vi "Open Calibration Files.vi"(0 "Pressure Calibration Path":path, 1 "Estimated Tube Gain":dbl, 5 "Flow Array Path":path, 7 "SPL Calibration Path":path, 9 "operation (0:open)":T1(ring), 11 "error in (no error)":errorcluster, 12 "access (0:read/write)":enum16{"read/write", "read-only", "write-only"}(ring)) -> (3 "Pressure Slope":dbl, 4 "Pressure Intercept":dbl, 6 "Flow Array":dbl[](array[numeric]), 8 "Microphone Sensitivity":dbl, 10 "SPL Gain":dbl, 15 "error out":errorcluster)   [LabVIEW 2020, in "CollectionSupport.lvlib"]
uses:
  CollectionSupport.lvlib
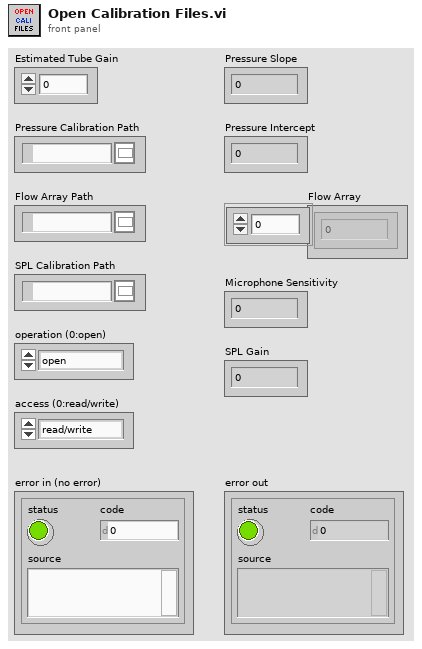
[diagram p1: front panel]
types:
  T1 = enum16{"open", "replace", "create", "open or create", "replace or create", "replace or create with confirmation"}
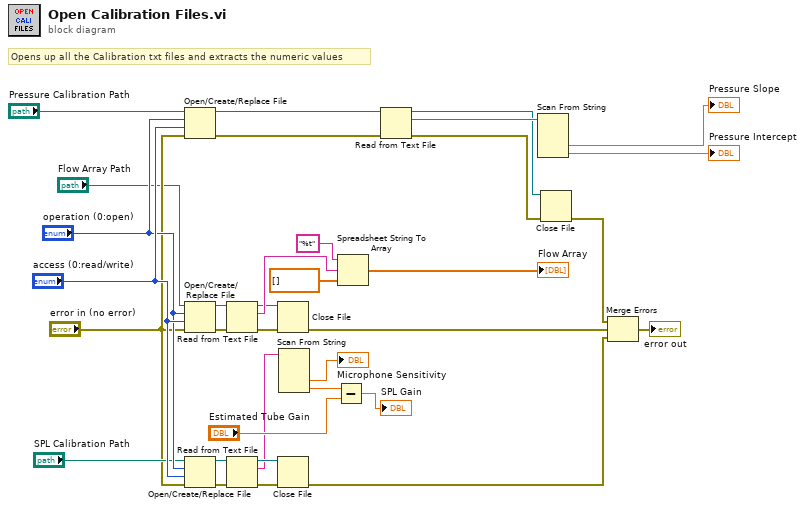
[diagram p0: block diagram]
diagram:
  # "Opens up all the Calibration txt files and extracts the numeric values"
  n1 = Open/Create/Replace File(file path (use dialog)="Pressure Calibration Path", error in="error in (no error)", operation (0:open)="operation (0:open)", access (0:read/write)="access (0:read/write)") -> (refnum out=w3:refnum<file>, error out=w1:errorcluster)  [unwired: 2 in, 1 out]
  n2 = Open/Create/Replace File(file path (use dialog)="Flow Array Path", error in="error in (no error)", operation (0:open)="operation (0:open)", access (0:read/write)="access (0:read/write)") -> (refnum out=w10:refnum<file>, error out=w8:errorcluster)  [unwired: 2 in, 1 out]
  n3 = Open/Create/Replace File(file path (use dialog)="SPL Calibration Path", error in="error in (no error)", operation (0:open)="operation (0:open)", access (0:read/write)="access (0:read/write)") -> (refnum out=w20:refnum<file>, error out=w22:errorcluster)  [unwired: 2 in, 1 out]
  n4 = Read from Text File(file (use dialog)=w10, error in=w8) -> (refnum out=w11:refnum<file>, text=w17:string, error out=w9:errorcluster)  [unwired: 2 in, 1 out]
  n5 = Read from Text File(file (use dialog)=w20, error in=w22) -> (refnum out=w28:refnum<file>, text=w27:string, error out=w23:errorcluster)  [unwired: 2 in, 1 out]
  n6 = Close File(refnum=w11, error in=w9) -> (error out=w15:errorcluster)  [unwired: 1 out]
  n7 = Close File(refnum=w28, error in=w23) -> (error out=w29:errorcluster)  [unwired: 1 out]
  n8 = Scan From String(input string=w27) -> (output 1=→"Microphone Sensitivity":dbl, output 2=w33:dbl)  [unwired: 5 in, 3 out]
  n9 = Subtract(x=w33, y="Estimated Tube Gain") -> (x-y=→"SPL Gain":dbl)
  n10 = Spreadsheet String To Array(format string="%t", spreadsheet string=w17, array type (2D Dbl)=dbl[] []) -> (array=→"Flow Array":dbl[])  [unwired: 1 in]
  n11 = Read from Text File(file (use dialog)=w3, error in=w1) -> (refnum out=w5:refnum<file>, text=w6:string, error out=w2:errorcluster)  [unwired: 2 in, 1 out]
  n12 = Scan From String "Scan From String"(input string=w6) -> (output 1=→"Pressure Slope":dbl, output 2=→"Pressure Intercept":dbl)  [unwired: 5 in, 3 out]
  n13 = Close File(refnum=w5, error in=w2) -> (error out=w14:errorcluster)  [unwired: 1 out]
  n14 = Merge Errors(w14, w15, w29) -> (→"error out":errorcluster)
